vi "Autonomous Independent.vi"() -> ()   [LabVIEW 2017]
doc: "This VI is called when autonomous begins, and will automatically be terminated when autonomous ends. You can carry out timed or sensor driven robot movement independently without needing to return to the caller."
uses:
  Control 1.ctl
  <vilib>/Rock Robotics/WPI/Solenoid/WPI_SolenoidValue.ctl
  <vilib>/Rock Robotics/Network Tables/NT Read String.vi
  <vilib>/Rock Robotics/WPI/Utilities/WPI_GetSetVariantRefNum.vi
  <vilib>/Rock Robotics/Network Tables/NT Write Numeric Array.vi
  <vilib>/Rock Robotics/WPI/RobotDrive/WPI_RobotDriveArcadeDrive_Standard(NoSaturation).vi
  <vilib>/Rock Robotics/WPI/Solenoid/WPI_SolenoidSetEnum.vi
panel:
  out "Current Movement, for debugging":T1 {"Y Joystick Value" scale=1.0..-1.0; "X Joystick Value" scale=-1.0..1.0}
  in  "Array of robot movements":T2(array[cluster])=[{"X Joystick Value"=0.39393939393939403, "Y Joystick Value"=0.0, "Delay (sec)"=1.0, "Movement Name"="turn"}, {"X Joystick Value"=-0.3737373737373737, "Y Joystick Value"=0.0, "Delay (sec)"=1.0, "Movement Name"="turn back"}] {"Y Joystick Value" scale=1.0..-1.0; "X Joystick Value" scale=-1.0..1.0}
  # "Be sure to right-click and choose Data Operations>>Make Current Value default if you want to save the array values with the VI"
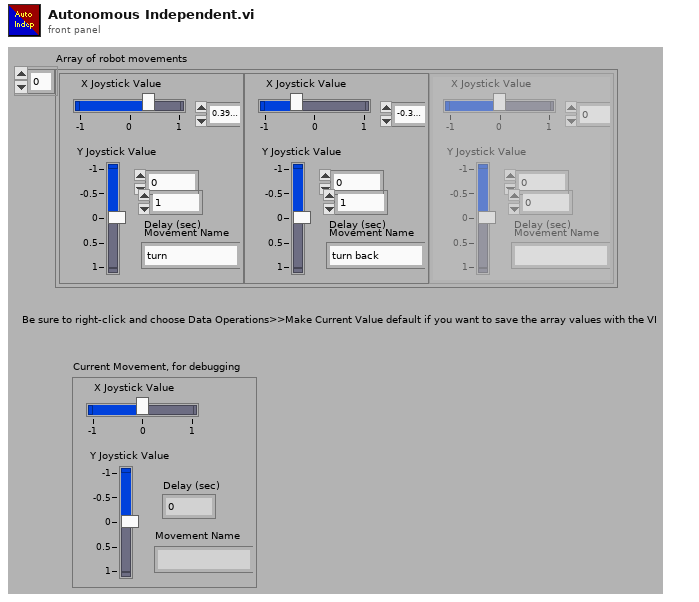
[diagram p1: front panel]
types:
  T1 = cluster{"X Joystick Value":dbl, "Y Joystick Value":dbl, "Delay (sec)":dbl, "Movement Name":string}
  T2 = cluster{"X Joystick Value":dbl, "Y Joystick Value":dbl, "Delay (sec)":dbl, "Movement Name":string}[]
  T3 = typedef "WPI_JoystickDevRef.ctl" = cluster{"Device":T4}
  T4 = typedef "WPI_JoystickDeviceEnum.ctl" = enum16{"USB 0", "USB 1", "USB 2", "USB 3", "USB 4", "USB 5"}
  T5 = typedef "Control 1.ctl" = dbl
  T6 = typedef "WPI_SolenoidValue.ctl" = enum16{"Off", "On", "Forward", "Reverse"}
  T7 = typedef "WPI_RobotDriveDevRef.ctl" = cluster{"DevStatus":errorcluster, "Motors[]":T8[], "Square Inputs":bool, "Max Output":dbl}
  T8 = typedef "WPI_MotorControlDeviceRef.ctl" = cluster{"DeviceStatus":errorcluster, "Type":T9, "PWM":cluster{"PWM Channel":T10, "DeadBand":T11}, "CAN":cluster{"Device Number":u8, "SetOutput VI Ref":variant, "GetOutput VI Ref":variant, "Enable VI Ref":variant, "Disable VI Ref":variant, "Data":variant}, "Invert":bool, "DIO PWM":cluster{"PWM \"Enable\" Channel":T10, "DIOChannel":T12, "PWM Rate":dbl}}
  T9 = typedef "WPI_MotorControlType.ctl" = enum16{"PWM", "CAN", "DIO PWM"}
  T10 = typedef "FPGA_DIOPWMChannel.ctl" = enum8{"PWM 0", "PWM 1", "PWM 2", "PWM 3", "PWM 4", "PWM 5", "PWM 6", "PWM 7", "PWM 8", "PWM 9", "PWM MXP 0", "PWM MXP 1", "PWM MXP 2", "PWM MXP 3", "PWM MXP 4", "PWM MXP 5", "PWM MXP 6", "PWM MXP 7", "PWM MXP 8", "PWM MXP 9", "Invalid"}
  T11 = typedef "WPI_PWMDeadband.ctl" = cluster{"Name":string, "maxPositivePwm":i32, "minPositivePwm":i32, "centerPwm":i32, "maxNegativePwm":i32, "minNegativePwm":i32, "angularRange":u16}
  T12 = typedef "FPGA_DIOChannel.ctl" = enum8{"DIO 0", "DIO 1", "DIO 2", "DIO 3", "DIO 4", "DIO 5", "DIO 6", "DIO 7", "DIO 8", "DIO 9", "DIO MXP 0", "DIO MXP 1", "DIO MXP 2", "DIO MXP 3", "DIO MXP 4", "DIO MXP 5", "DIO MXP 6", "DIO MXP 7", "DIO MXP 8", "DIO MXP 9", "DIO MXP 10", "DIO MXP 11", "DIO MXP 12", "DIO MXP 13", "DIO MXP 14", "DIO MXP 15", "SPI Port CS1", "SPI Port CS2", "SPI Port CS3", "SPI Port MISO", "SPI Port MOSI", "Invalid"}
  T13 = typedef "WPI_SolenoidDevRef.ctl" = cluster{"DevStatus":errorcluster, "Pneumatics Control Module":u8, "Forward Solenoid Channel":T14, "Reverse Solenoid Channel":T14}
  T14 = typedef "WPI_SolenoidChannel.ctl" = enum8{"Solenoid 0", "Solenoid 1", "Solenoid 2", "Solenoid 3", "Solenoid 4", "Solenoid 5", "Solenoid 6", "Solenoid 7", "Invalid"}
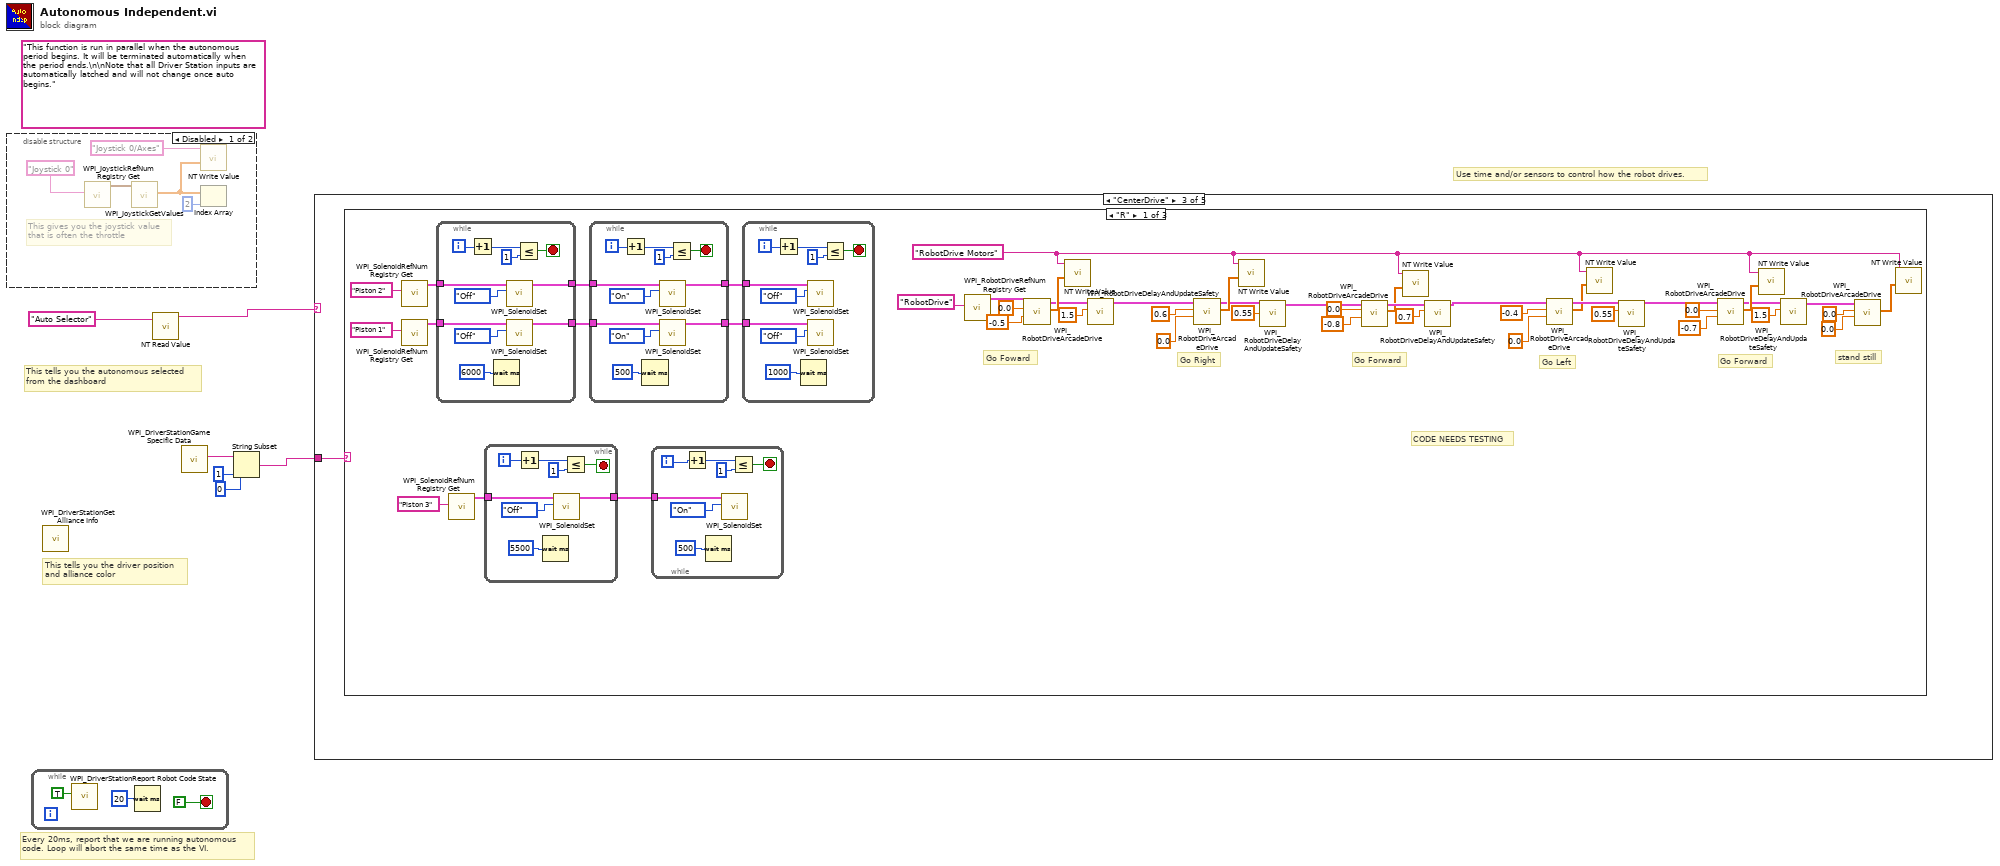
[diagram p0: block diagram]
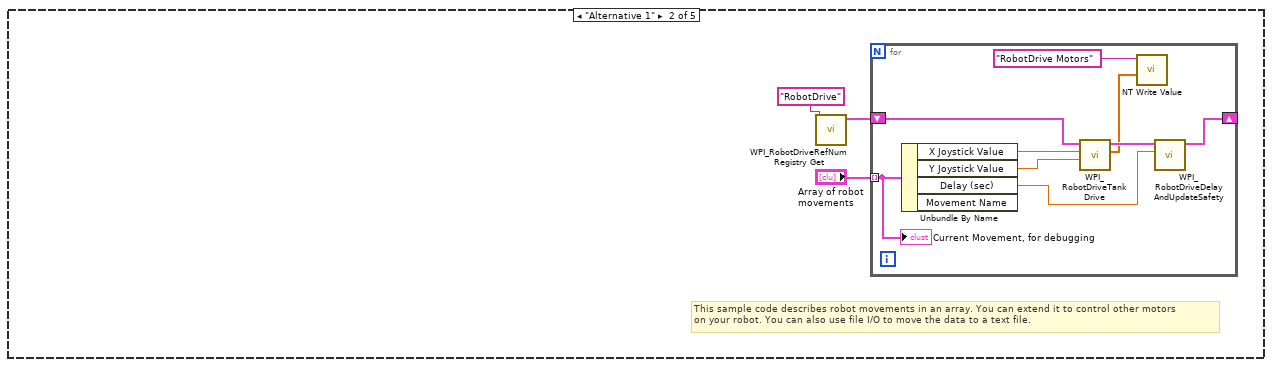
[diagram p4: hidden frame]
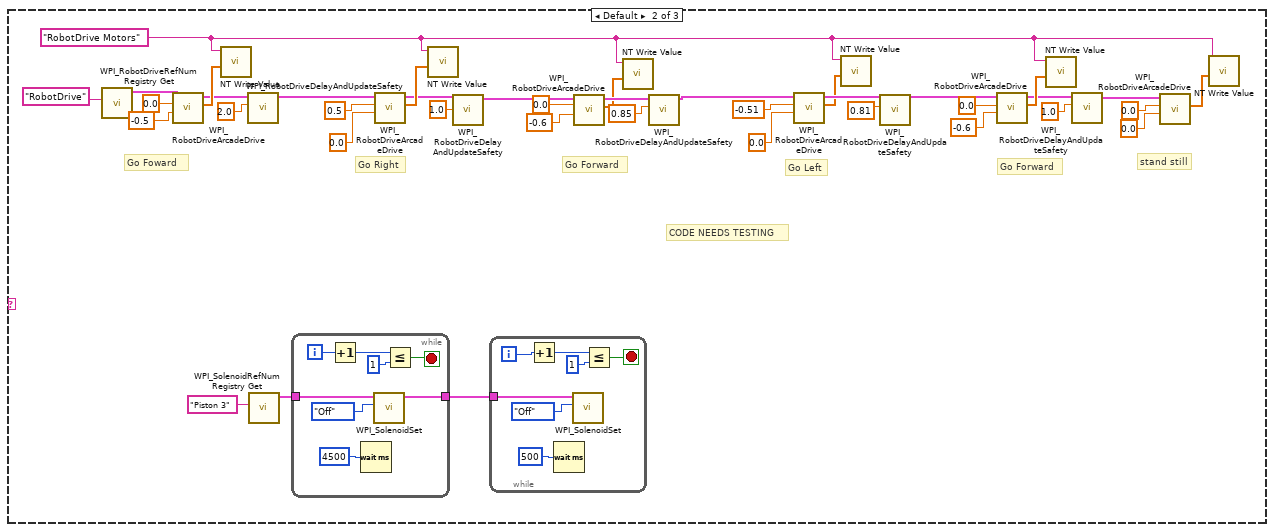
[diagram p5: hidden frame]
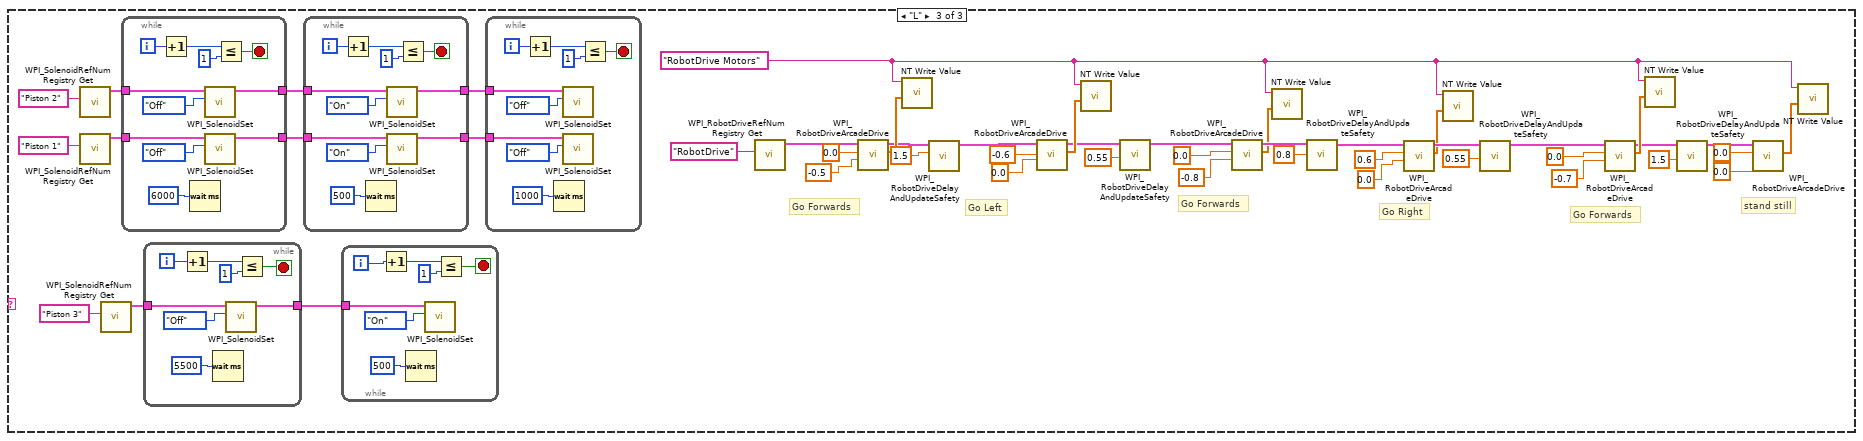
[diagram p6: hidden frame]
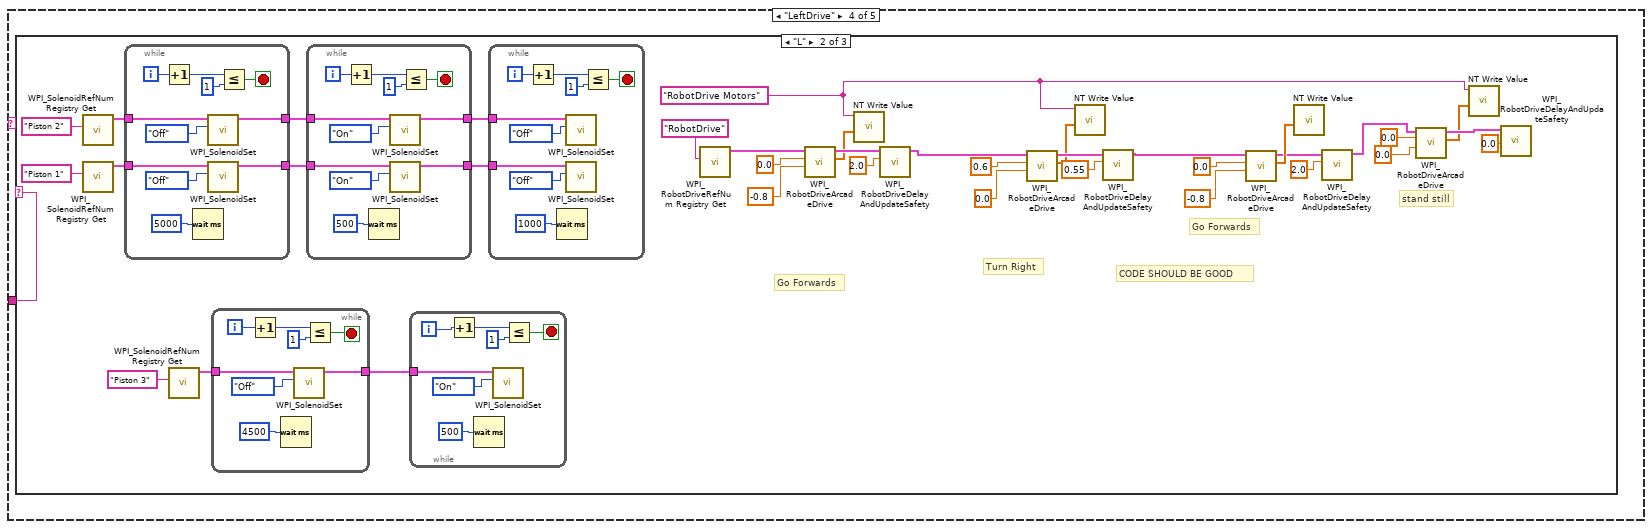
[diagram p7: hidden frame]
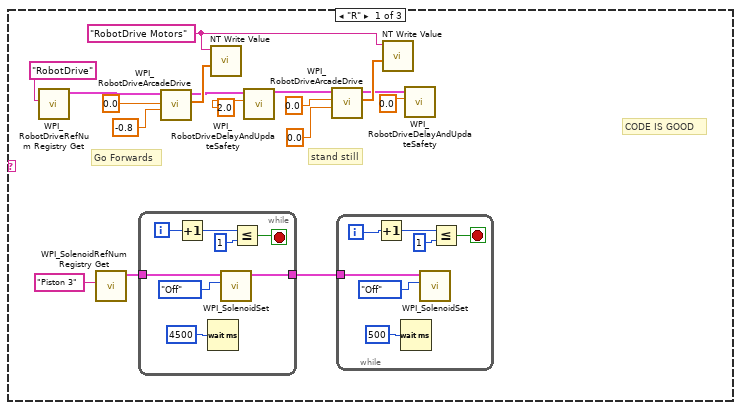
[diagram p8: hidden frame]
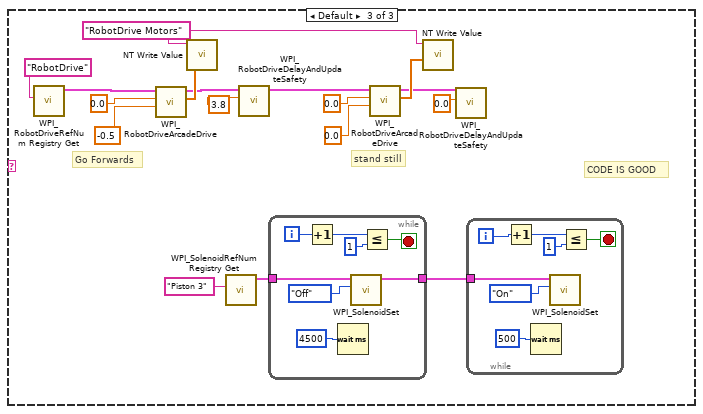
[diagram p9: hidden frame]
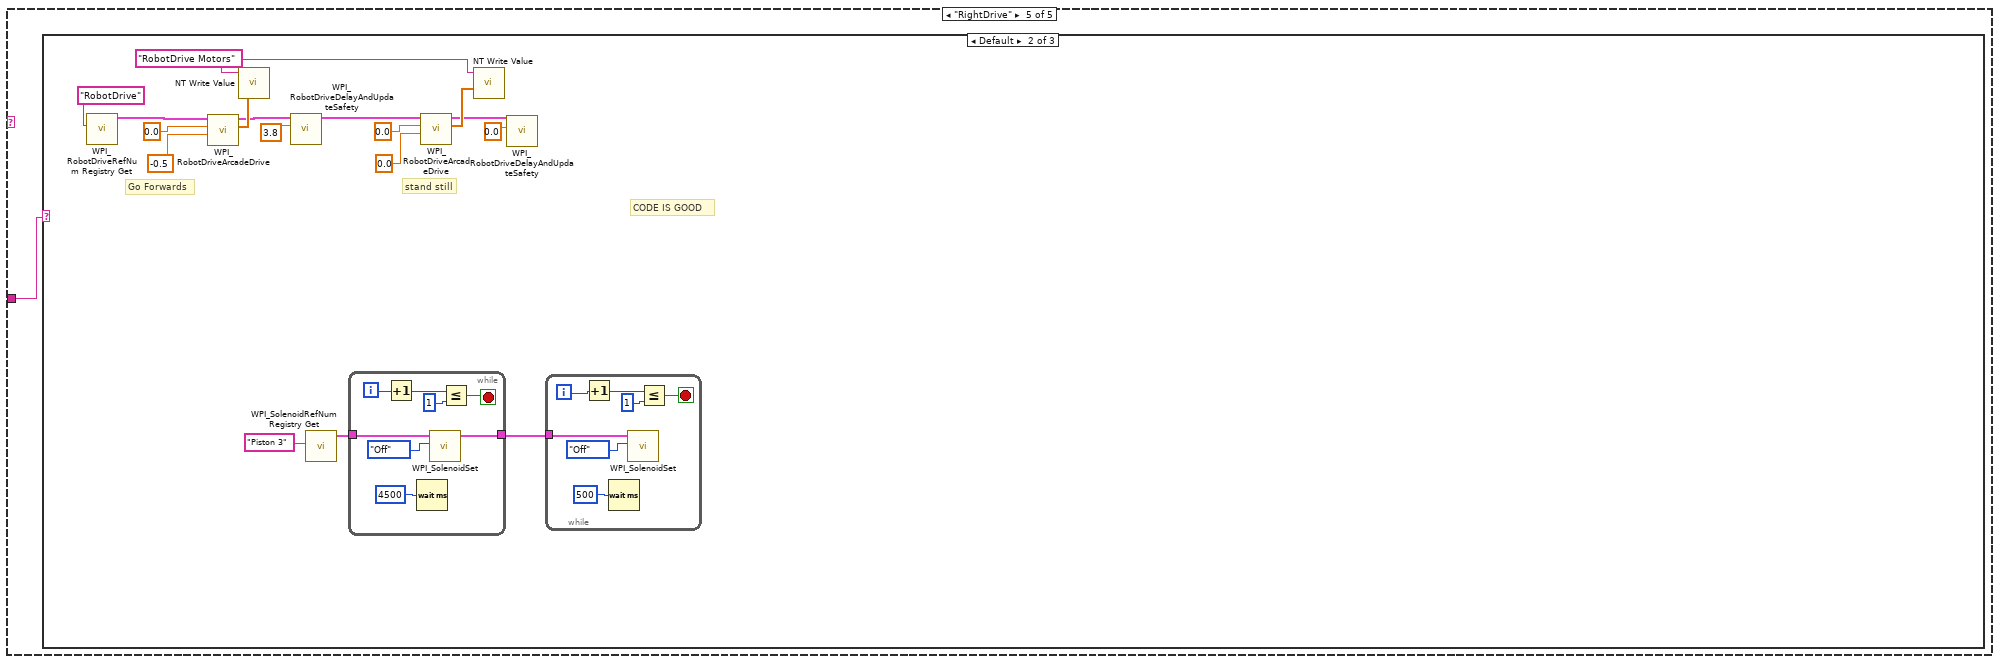
[diagram p10: hidden frame]
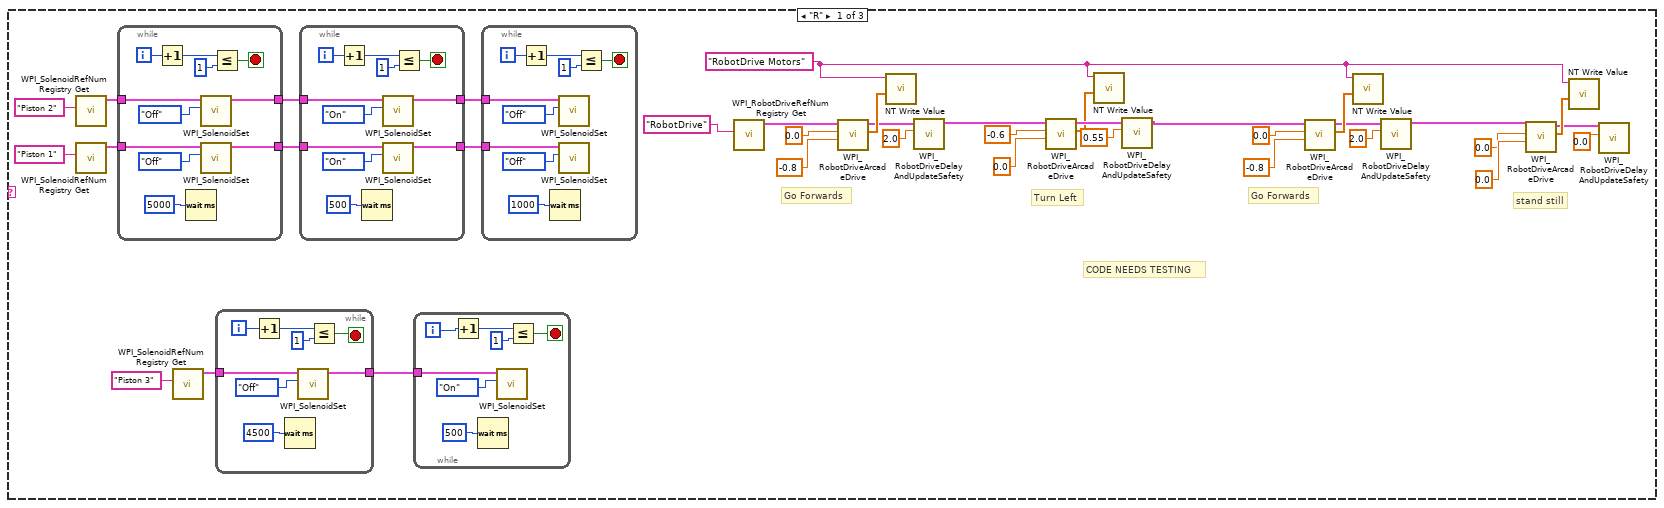
[diagram p11: hidden frame]
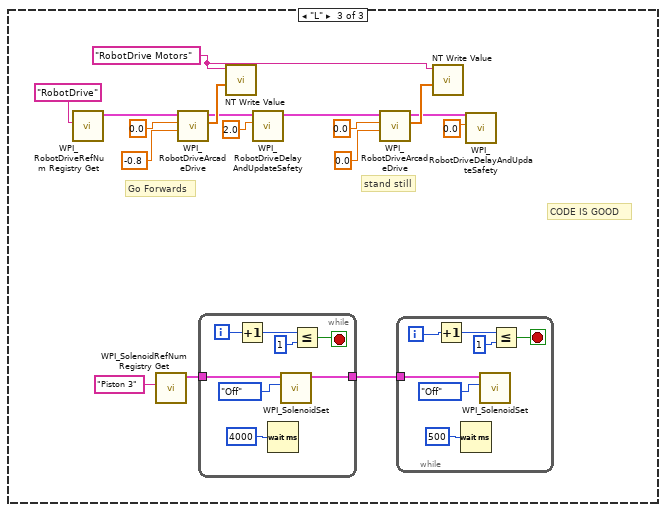
[diagram p12: hidden frame]
diagram:
  (unwired) "This function is run in parallel when the autonomous period begins. It will be terminated automatically when the period ends.\n\nNote that all Driver Station inputs are automatically latched and will not change once auto begins."
  # "This tells you the autonomous selected\nfrom the dashboard"
  # "Every 20ms, report that we are running autonomous\ncode. Loop will abort the same time as the VI."
  # "Use time and/or sensors to control how the robot drives."
  # "This tells you the driver position\nand alliance color"
  n1 = disable-structure shown="Disabled" {
    frame Disabled {
      # "This gives you the joystick value\nthat is often the throttle"
      n2 = call <vilib>:"WPI_JoystickRefNum Registry Get.vi"("refnum name"="Joystick 0") -> ("JoystickDevRef"=w10:T3)  [unwired: 1 in, 9 out]
      n3 = call <vilib>:"WPI_JoystickGetValues.vi"("JoystickDevRef"=w10) -> ("Axes"=w8:dbl[])  [unwired: 6 in, 4 out]
      n4 = call-poly <vilib>:"NT Write Value.vi"("Numeric Array"=w8, "Name"="Joystick 0/Axes") -> ()  [unwired: 9 in, 1 out]
      n5 = Index Array(array=w8, index=2) -> ()  [unwired: 1 out]
    }
    frame Enabled {
    }
  }
  n6 = while {
    stop <- FALSE stop-if-true
    n7 = call <vilib>:"WPI_DriverStationReport Robot Code State.vi"("Autonomous"=TRUE) -> ()  [unwired: 10 in, 1 out]
    n8 = Wait (ms)(milliseconds to wait=u32 20) -> ()  [unwired: 1 out]
  }
  n9 = call <vilib>:"WPI_DriverStationGet Alliance Info.vi"() -> ()  [unwired: 12 out]
  n10 = call-poly <vilib>:"NT Read Value.vi"("Name"="Auto Selector") -> ("String"=w5:string)  [unwired: 9 in, 1 out]
  n11 = call <vilib>:"WPI_DriverStationGame Specific Data.vi"() -> ("Game Specific Data"=w4:string)  [unwired: 11 in]
  n12 = String Subset(string=w4, offset (0)=0, length (rest)=1) -> (substring=w2:string)
  n13 = case shown="\"CenterDrive\"" w5 {
    tunnel: w2 -> [_ _ w27 w268 w416]
    frame Default {
      # "You can put your main auto here, or you can right-click on the case and make any\nother frame be the default case."
      # "This is the frame that will execute if no selection is made, or if it is not recognized"
    }
    frame "Alternative 1" {
      # "This sample code describes robot movements in an array. You can extend it to control other motors\non your robot. You can also use file I/O to move the data to a text file."
      n14 = call <vilib>:"WPI_RobotDriveRefNum Registry Get.vi"("refnum name"="RobotDrive") -> ("RobotDriveDevRef"=w16:T7)  [unwired: 1 in, 9 out]
      n15 = for {
        shift-right: [w24] -> _
        shift-left: w16 -> [w25]
        tunnel: "Array of robot movements" -> [w20] mode=indexing
        n16 = Unbundle By Name(w20) -> ("X Joystick Value"=w23:dbl, "Y Joystick Value"=w22:dbl, "Delay (sec)"=w21:dbl)  [unwired: 1 out]
        n17 = call <vilib>:"WPI_RobotDriveTankDrive.vi"("Right axis value"=w22, "Left axis value"=w23, "RobotDriveDevRef"=w25) -> ("Motor Values"=w18:dbl[], "RobotDriveDevRef"=w26:T7)  [unwired: 6 in, 1 out]
        n18 = call-poly <vilib>:"NT Write Value.vi"("Numeric Array"=w18, "Name"="RobotDrive Motors") -> ()  [unwired: 9 in, 1 out]
        n19 = call <vilib>:"WPI_RobotDriveDelayAndUpdateSafety.vi"("Delay (s)"=w21, "RobotDriveDevRef"=w26) -> ("RobotDriveDevRef 2"=w24:T7)  [unwired: 8 in, 1 out]
        "Current Movement, for debugging" <- w20
      }
    }
    frame "CenterDrive" {
      n20 = case shown="\"R\"" w27 {
        frame "R" {
          w39 = "RobotDrive Motors" ("Name")
          # "CODE NEEDS TESTING"
          # "Go Forward"
          # "Go Left"
          # "Go Forward"
          # "stand still"
          # "Go Right"
          # "Go Foward"
          n21 = call <vilib>:"WPI_SolenoidRefNum Registry Get.vi"("refnum name"="Piston 2") -> ("SolenoidDevRef"=w36:T13)  [unwired: 9 in, 1 out]
          n22 = call <vilib>:"WPI_SolenoidRefNum Registry Get.vi"("refnum name"="Piston 1") -> ("SolenoidDevRef"=w35:T13)  [unwired: 9 in, 1 out]
          n23 = while {
            tunnel: w36 -> [w114]
            tunnel: w35 -> [w112]
            tunnel: [w111] -> w34
            tunnel: [w110] -> w33
            i -> [w120]
            stop <- w118 stop-if-true
            n24 = Increment(x=w120) -> (x+1=w119:i32)
            n25 = Wait (ms)(milliseconds to wait=u32 6000) -> ()  [unwired: 1 out]
            n26 = call-poly <vilib>:"WPI_SolenoidSet.vi"("Value"=WPI_SolenoidValue."Off", "SolenoidDevRef"=w114) -> ("SolenoidDevRef"=w111:T13)  [unwired: 8 in, 1 out]
            n27 = call-poly <vilib>:"WPI_SolenoidSet.vi"("Value"=WPI_SolenoidValue."Off", "SolenoidDevRef"=w112) -> ("SolenoidDevRef"=w110:T13)  [unwired: 8 in, 1 out]
            n28 = Less Or Equal?(x=w119, y=1) -> (x <= y?=w118:bool)
          }
          n29 = call <vilib>:"WPI_SolenoidRefNum Registry Get.vi"("refnum name"="Piston 3") -> ("SolenoidDevRef"=w29:T13)  [unwired: 9 in, 1 out]
          n30 = while {
            tunnel: w29 -> [w83]
            tunnel: [w82] -> w28
            i -> [w84]
            stop <- w85 stop-if-true
            n31 = Increment(x=w84) -> (x+1=w86:i32)
            n32 = Wait (ms)(milliseconds to wait=u32 5500) -> ()  [unwired: 1 out]
            n33 = call-poly <vilib>:"WPI_SolenoidSet.vi"("Value"=WPI_SolenoidValue."Off", "SolenoidDevRef"=w83) -> ("SolenoidDevRef"=w82:T13)  [unwired: 8 in, 1 out]
            n34 = Less Or Equal?(x=w86, y=1) -> (x <= y?=w85:bool)
          }
          n35 = while {
            tunnel: w34 -> [w102]
            tunnel: w33 -> [w101]
            tunnel: [w100] -> w32
            tunnel: [w99] -> w31
            i -> [w106]
            stop <- w105 stop-if-true
            n36 = Increment(x=w106) -> (x+1=w107:i32)
            n37 = Wait (ms)(milliseconds to wait=u32 500) -> ()  [unwired: 1 out]
            n38 = call-poly <vilib>:"WPI_SolenoidSet.vi"("Value"=WPI_SolenoidValue."On", "SolenoidDevRef"=w102) -> ("SolenoidDevRef"=w99:T13)  [unwired: 8 in, 1 out]
            n39 = call-poly <vilib>:"WPI_SolenoidSet.vi"("Value"=WPI_SolenoidValue."On", "SolenoidDevRef"=w101) -> ("SolenoidDevRef"=w100:T13)  [unwired: 8 in, 1 out]
            n40 = Less Or Equal?(x=w107, y=1) -> (x <= y?=w105:bool)
          }
          n41 = while {
            tunnel: w28 -> [w75]
            i -> [w76]
            stop <- w77 stop-if-true
            n42 = Increment(x=w76) -> (x+1=w80:i32)
            n43 = Wait (ms)(milliseconds to wait=u32 500) -> ()  [unwired: 1 out]
            n44 = call-poly <vilib>:"WPI_SolenoidSet.vi"("Value"=WPI_SolenoidValue."On", "SolenoidDevRef"=w75) -> ()  [unwired: 8 in, 2 out]
            n45 = Less Or Equal?(x=w80, y=1) -> (x <= y?=w77:bool)
          }
          n46 = while {
            tunnel: w32 -> [w91]
            tunnel: w31 -> [w90]
            i -> [w95]
            stop <- w94 stop-if-true
            n47 = Increment(x=w95) -> (x+1=w96:i32)
            n48 = Wait (ms)(milliseconds to wait=u32 1000) -> ()  [unwired: 1 out]
            n49 = call-poly <vilib>:"WPI_SolenoidSet.vi"("Value"=WPI_SolenoidValue."Off", "SolenoidDevRef"=w90) -> ()  [unwired: 8 in, 2 out]
            n50 = call-poly <vilib>:"WPI_SolenoidSet.vi"("Value"=WPI_SolenoidValue."Off", "SolenoidDevRef"=w91) -> ()  [unwired: 8 in, 2 out]
            n51 = Less Or Equal?(x=w96, y=1) -> (x <= y?=w94:bool)
          }
          n52 = call <vilib>:"WPI_RobotDriveRefNum Registry Get.vi"("refnum name"="RobotDrive") -> ("RobotDriveDevRef"=w68:T7)  [unwired: 1 in, 9 out]
          n53 = call-poly <vilib>:"WPI_RobotDriveArcadeDrive.vi"("Y axis value"=-0.5 ("X axis value"), "X axis value"=0.0, "RobotDriveDevRef"=w68) -> ("Motor Values"=w74:dbl[], "RobotDriveDevRef"=w71:T7)  [unwired: 6 in, 1 out]
          n54 = call-poly <vilib>:"NT Write Value.vi"("Numeric Array"=w74, "Name"=w39) -> ()  [unwired: 9 in, 1 out]
          n55 = call <vilib>:"WPI_RobotDriveDelayAndUpdateSafety.vi"("Delay (s)"=T5 1.5, "RobotDriveDevRef"=w71) -> ("RobotDriveDevRef 2"=w70:T7)  [unwired: 8 in, 1 out]
          n56 = call-poly <vilib>:"WPI_RobotDriveArcadeDrive.vi"("Y axis value"=0.0 ("X axis value"), "X axis value"=0.6, "RobotDriveDevRef"=w70) -> ("Motor Values"=w73:dbl[], "RobotDriveDevRef"=w69:T7)  [unwired: 6 in, 1 out]
          n57 = call-poly <vilib>:"NT Write Value.vi"("Numeric Array"=w73, "Name"=w39) -> ()  [unwired: 9 in, 1 out]
          n58 = call <vilib>:"WPI_RobotDriveDelayAndUpdateSafety.vi"("Delay (s)"=0.55, "RobotDriveDevRef"=w69) -> ("RobotDriveDevRef 2"=w54:T7)  [unwired: 8 in, 1 out]
          n59 = call-poly <vilib>:"WPI_RobotDriveArcadeDrive.vi"("Y axis value"=-0.8 ("X axis value"), "X axis value"=0.0, "RobotDriveDevRef"=w54) -> ("Motor Values"=w55:dbl[], "RobotDriveDevRef"=w56:T7)  [unwired: 6 in, 1 out]
          n60 = call-poly <vilib>:"NT Write Value.vi"("Numeric Array"=w55, "Name"=w39) -> ()  [unwired: 9 in, 1 out]
          n61 = call <vilib>:"WPI_RobotDriveDelayAndUpdateSafety.vi"("Delay (s)"=T5 0.7, "RobotDriveDevRef"=w56) -> ("RobotDriveDevRef 2"=w48:T7)  [unwired: 8 in, 1 out]
          n62 = call-poly <vilib>:"WPI_RobotDriveArcadeDrive.vi"("Y axis value"=0.0 ("X axis value"), "X axis value"=-0.4, "RobotDriveDevRef"=w48) -> ("Motor Values"=w49:dbl[], "RobotDriveDevRef"=w50:T7)  [unwired: 6 in, 1 out]
          n63 = call-poly <vilib>:"NT Write Value.vi"("Numeric Array"=w49, "Name"=w39) -> ()  [unwired: 9 in, 1 out]
          n64 = call <vilib>:"WPI_RobotDriveDelayAndUpdateSafety.vi"("Delay (s)"=0.55, "RobotDriveDevRef"=w50) -> ("RobotDriveDevRef 2"=w42:T7)  [unwired: 8 in, 1 out]
          n65 = call-poly <vilib>:"WPI_RobotDriveArcadeDrive.vi"("Y axis value"=-0.7 ("X axis value"), "X axis value"=0.0, "RobotDriveDevRef"=w42) -> ("Motor Values"=w47:dbl[], "RobotDriveDevRef"=w46:T7)  [unwired: 6 in, 1 out]
          n66 = call-poly <vilib>:"NT Write Value.vi"("Numeric Array"=w47, "Name"=w39) -> ()  [unwired: 9 in, 1 out]
          n67 = call <vilib>:"WPI_RobotDriveDelayAndUpdateSafety.vi"("Delay (s)"=T5 1.5, "RobotDriveDevRef"=w46) -> ("RobotDriveDevRef 2"=w41:T7)  [unwired: 8 in, 1 out]
          n68 = call-poly <vilib>:"WPI_RobotDriveArcadeDrive.vi"("Y axis value"=0.0 ("X axis value"), "X axis value"=0.0, "RobotDriveDevRef"=w41) -> ("Motor Values"=w72:dbl[])  [unwired: 6 in, 2 out]
          n69 = call-poly <vilib>:"NT Write Value.vi"("Numeric Array"=w72, "Name"=w39) -> ()  [unwired: 9 in, 1 out]
        }
        frame Default {
          w124 = "RobotDrive Motors" ("Name")
          # "CODE NEEDS TESTING"
          # "Go Forward"
          # "Go Left"
          # "Go Forward"
          # "stand still"
          # "Go Right"
          # "Go Foward"
          n70 = call <vilib>:"WPI_RobotDriveRefNum Registry Get.vi"("refnum name"="RobotDrive") -> ("RobotDriveDevRef"=w153:T7)  [unwired: 1 in, 9 out]
          n71 = call-poly <vilib>:"WPI_RobotDriveArcadeDrive.vi"("Y axis value"=-0.5 ("X axis value"), "X axis value"=0.0, "RobotDriveDevRef"=w153) -> ("Motor Values"=w159:dbl[], "RobotDriveDevRef"=w156:T7)  [unwired: 6 in, 1 out]
          n72 = call-poly <vilib>:"NT Write Value.vi"("Numeric Array"=w159, "Name"=w124) -> ()  [unwired: 9 in, 1 out]
          n73 = call <vilib>:"WPI_RobotDriveDelayAndUpdateSafety.vi"("Delay (s)"=T5 2.0, "RobotDriveDevRef"=w156) -> ("RobotDriveDevRef 2"=w155:T7)  [unwired: 8 in, 1 out]
          n74 = call <vilib>:"WPI_SolenoidRefNum Registry Get.vi"("refnum name"="Piston 3") -> ("SolenoidDevRef"=w122:T13)  [unwired: 9 in, 1 out]
          n75 = while {
            tunnel: w122 -> [w168]
            tunnel: [w167] -> w121
            i -> [w169]
            stop <- w170 stop-if-true
            n76 = Increment(x=w169) -> (x+1=w171:i32)
            n77 = Wait (ms)(milliseconds to wait=u32 4500) -> ()  [unwired: 1 out]
            n78 = call-poly <vilib>:"WPI_SolenoidSet.vi"("Value"=WPI_SolenoidValue."Off", "SolenoidDevRef"=w168) -> ("SolenoidDevRef"=w167:T13)  [unwired: 8 in, 1 out]
            n79 = Less Or Equal?(x=w171, y=1) -> (x <= y?=w170:bool)
          }
          n80 = call-poly <vilib>:"WPI_RobotDriveArcadeDrive.vi"("Y axis value"=0.0 ("X axis value"), "X axis value"=0.5, "RobotDriveDevRef"=w155) -> ("Motor Values"=w158:dbl[], "RobotDriveDevRef"=w154:T7)  [unwired: 6 in, 1 out]
          n81 = call-poly <vilib>:"NT Write Value.vi"("Numeric Array"=w158, "Name"=w124) -> ()  [unwired: 9 in, 1 out]
          n82 = call <vilib>:"WPI_RobotDriveDelayAndUpdateSafety.vi"("Delay (s)"=1.0, "RobotDriveDevRef"=w154) -> ("RobotDriveDevRef 2"=w139:T7)  [unwired: 8 in, 1 out]
          n83 = while {
            tunnel: w121 -> [w160]
            i -> [w161]
            stop <- w162 stop-if-true
            n84 = Increment(x=w161) -> (x+1=w165:i32)
            n85 = Wait (ms)(milliseconds to wait=u32 500) -> ()  [unwired: 1 out]
            n86 = call-poly <vilib>:"WPI_SolenoidSet.vi"("Value"=WPI_SolenoidValue."Off", "SolenoidDevRef"=w160) -> ()  [unwired: 8 in, 2 out]
            n87 = Less Or Equal?(x=w165, y=1) -> (x <= y?=w162:bool)
          }
          n88 = call-poly <vilib>:"WPI_RobotDriveArcadeDrive.vi"("Y axis value"=-0.6 ("X axis value"), "X axis value"=0.0, "RobotDriveDevRef"=w139) -> ("Motor Values"=w140:dbl[], "RobotDriveDevRef"=w141:T7)  [unwired: 6 in, 1 out]
          n89 = call-poly <vilib>:"NT Write Value.vi"("Numeric Array"=w140, "Name"=w124) -> ()  [unwired: 9 in, 1 out]
          n90 = call <vilib>:"WPI_RobotDriveDelayAndUpdateSafety.vi"("Delay (s)"=T5 0.85, "RobotDriveDevRef"=w141) -> ("RobotDriveDevRef 2"=w133:T7)  [unwired: 8 in, 1 out]
          n91 = call-poly <vilib>:"WPI_RobotDriveArcadeDrive.vi"("Y axis value"=0.0 ("X axis value"), "X axis value"=-0.51, "RobotDriveDevRef"=w133) -> ("Motor Values"=w134:dbl[], "RobotDriveDevRef"=w135:T7)  [unwired: 6 in, 1 out]
          n92 = call-poly <vilib>:"NT Write Value.vi"("Numeric Array"=w134, "Name"=w124) -> ()  [unwired: 9 in, 1 out]
          n93 = call <vilib>:"WPI_RobotDriveDelayAndUpdateSafety.vi"("Delay (s)"=0.81, "RobotDriveDevRef"=w135) -> ("RobotDriveDevRef 2"=w127:T7)  [unwired: 8 in, 1 out]
          n94 = call-poly <vilib>:"WPI_RobotDriveArcadeDrive.vi"("Y axis value"=-0.6 ("X axis value"), "X axis value"=0.0, "RobotDriveDevRef"=w127) -> ("Motor Values"=w132:dbl[], "RobotDriveDevRef"=w131:T7)  [unwired: 6 in, 1 out]
          n95 = call-poly <vilib>:"NT Write Value.vi"("Numeric Array"=w132, "Name"=w124) -> ()  [unwired: 9 in, 1 out]
          n96 = call <vilib>:"WPI_RobotDriveDelayAndUpdateSafety.vi"("Delay (s)"=T5 1.0, "RobotDriveDevRef"=w131) -> ("RobotDriveDevRef 2"=w126:T7)  [unwired: 8 in, 1 out]
          n97 = call-poly <vilib>:"WPI_RobotDriveArcadeDrive.vi"("Y axis value"=0.0 ("X axis value"), "X axis value"=0.0, "RobotDriveDevRef"=w126) -> ("Motor Values"=w157:dbl[])  [unwired: 6 in, 2 out]
          n98 = call-poly <vilib>:"NT Write Value.vi"("Numeric Array"=w157, "Name"=w124) -> ()  [unwired: 9 in, 1 out]
        }
        frame "L" {
          w186 = "RobotDrive Motors" ("Name")
          # "Go Forwards"
          # "Go Right"
          # "Go Forwards"
          # "stand still"
          # "Go Left"
          # "Go Forwards"
          n99 = call <vilib>:"WPI_SolenoidRefNum Registry Get.vi"("refnum name"="Piston 2") -> ("SolenoidDevRef"=w183:T13)  [unwired: 9 in, 1 out]
          n100 = call <vilib>:"WPI_SolenoidRefNum Registry Get.vi"("refnum name"="Piston 1") -> ("SolenoidDevRef"=w182:T13)  [unwired: 9 in, 1 out]
          n101 = call <vilib>:"WPI_SolenoidRefNum Registry Get.vi"("refnum name"="Piston 3") -> ("SolenoidDevRef"=w176:T13)  [unwired: 9 in, 1 out]
          n102 = while {
            tunnel: w183 -> [w261]
            tunnel: w182 -> [w259]
            tunnel: [w258] -> w181
            tunnel: [w257] -> w180
            i -> [w267]
            stop <- w265 stop-if-true
            n103 = Increment(x=w267) -> (x+1=w266:i32)
            n104 = Wait (ms)(milliseconds to wait=u32 6000) -> ()  [unwired: 1 out]
            n105 = call-poly <vilib>:"WPI_SolenoidSet.vi"("Value"=WPI_SolenoidValue."Off", "SolenoidDevRef"=w261) -> ("SolenoidDevRef"=w258:T13)  [unwired: 8 in, 1 out]
            n106 = call-poly <vilib>:"WPI_SolenoidSet.vi"("Value"=WPI_SolenoidValue."Off", "SolenoidDevRef"=w259) -> ("SolenoidDevRef"=w257:T13)  [unwired: 8 in, 1 out]
            n107 = Less Or Equal?(x=w266, y=1) -> (x <= y?=w265:bool)
          }
          n108 = while {
            tunnel: w176 -> [w230]
            tunnel: [w229] -> w175
            i -> [w231]
            stop <- w232 stop-if-true
            n109 = Increment(x=w231) -> (x+1=w233:i32)
            n110 = Wait (ms)(milliseconds to wait=u32 5500) -> ()  [unwired: 1 out]
            n111 = call-poly <vilib>:"WPI_SolenoidSet.vi"("Value"=WPI_SolenoidValue."Off", "SolenoidDevRef"=w230) -> ("SolenoidDevRef"=w229:T13)  [unwired: 8 in, 1 out]
            n112 = Less Or Equal?(x=w233, y=1) -> (x <= y?=w232:bool)
          }
          n113 = while {
            tunnel: w181 -> [w249]
            tunnel: w180 -> [w248]
            tunnel: [w247] -> w179
            tunnel: [w246] -> w178
            i -> [w253]
            stop <- w252 stop-if-true
            n114 = Increment(x=w253) -> (x+1=w254:i32)
            n115 = Wait (ms)(milliseconds to wait=u32 500) -> ()  [unwired: 1 out]
            n116 = call-poly <vilib>:"WPI_SolenoidSet.vi"("Value"=WPI_SolenoidValue."On", "SolenoidDevRef"=w249) -> ("SolenoidDevRef"=w246:T13)  [unwired: 8 in, 1 out]
            n117 = call-poly <vilib>:"WPI_SolenoidSet.vi"("Value"=WPI_SolenoidValue."On", "SolenoidDevRef"=w248) -> ("SolenoidDevRef"=w247:T13)  [unwired: 8 in, 1 out]
            n118 = Less Or Equal?(x=w254, y=1) -> (x <= y?=w252:bool)
          }
          n119 = while {
            tunnel: w175 -> [w222]
            i -> [w223]
            stop <- w224 stop-if-true
            n120 = Increment(x=w223) -> (x+1=w227:i32)
            n121 = Wait (ms)(milliseconds to wait=u32 500) -> ()  [unwired: 1 out]
            n122 = call-poly <vilib>:"WPI_SolenoidSet.vi"("Value"=WPI_SolenoidValue."On", "SolenoidDevRef"=w222) -> ()  [unwired: 8 in, 2 out]
            n123 = Less Or Equal?(x=w227, y=1) -> (x <= y?=w224:bool)
          }
          n124 = while {
            tunnel: w179 -> [w238]
            tunnel: w178 -> [w237]
            i -> [w242]
            stop <- w241 stop-if-true
            n125 = Increment(x=w242) -> (x+1=w243:i32)
            n126 = Wait (ms)(milliseconds to wait=u32 1000) -> ()  [unwired: 1 out]
            n127 = call-poly <vilib>:"WPI_SolenoidSet.vi"("Value"=WPI_SolenoidValue."Off", "SolenoidDevRef"=w237) -> ()  [unwired: 8 in, 2 out]
            n128 = call-poly <vilib>:"WPI_SolenoidSet.vi"("Value"=WPI_SolenoidValue."Off", "SolenoidDevRef"=w238) -> ()  [unwired: 8 in, 2 out]
            n129 = Less Or Equal?(x=w243, y=1) -> (x <= y?=w241:bool)
          }
          n130 = call <vilib>:"WPI_RobotDriveRefNum Registry Get.vi"("refnum name"="RobotDrive") -> ("RobotDriveDevRef"=w215:T7)  [unwired: 1 in, 9 out]
          n131 = call-poly <vilib>:"WPI_RobotDriveArcadeDrive.vi"("Y axis value"=-0.5 ("X axis value"), "X axis value"=0.0, "RobotDriveDevRef"=w215) -> ("Motor Values"=w221:dbl[], "RobotDriveDevRef"=w218:T7)  [unwired: 6 in, 1 out]
          n132 = call-poly <vilib>:"NT Write Value.vi"("Numeric Array"=w221, "Name"=w186) -> ()  [unwired: 9 in, 1 out]
          n133 = call <vilib>:"WPI_RobotDriveDelayAndUpdateSafety.vi"("Delay (s)"=T5 1.5, "RobotDriveDevRef"=w218) -> ("RobotDriveDevRef 2"=w217:T7)  [unwired: 8 in, 1 out]
          n134 = call-poly <vilib>:"WPI_RobotDriveArcadeDrive.vi"("Y axis value"=0.0 ("X axis value"), "X axis value"=-0.6, "RobotDriveDevRef"=w217) -> ("Motor Values"=w220:dbl[], "RobotDriveDevRef"=w216:T7)  [unwired: 6 in, 1 out]
          n135 = call-poly <vilib>:"NT Write Value.vi"("Numeric Array"=w220, "Name"=w186) -> ()  [unwired: 9 in, 1 out]
          n136 = call <vilib>:"WPI_RobotDriveDelayAndUpdateSafety.vi"("Delay (s)"=0.55, "RobotDriveDevRef"=w216) -> ("RobotDriveDevRef 2"=w201:T7)  [unwired: 8 in, 1 out]
          n137 = call-poly <vilib>:"WPI_RobotDriveArcadeDrive.vi"("Y axis value"=-0.8 ("X axis value"), "X axis value"=0.0, "RobotDriveDevRef"=w201) -> ("Motor Values"=w202:dbl[], "RobotDriveDevRef"=w203:T7)  [unwired: 6 in, 1 out]
          n138 = call-poly <vilib>:"NT Write Value.vi"("Numeric Array"=w202, "Name"=w186) -> ()  [unwired: 9 in, 1 out]
          n139 = call <vilib>:"WPI_RobotDriveDelayAndUpdateSafety.vi"("Delay (s)"=T5 0.8, "RobotDriveDevRef"=w203) -> ("RobotDriveDevRef 2"=w195:T7)  [unwired: 8 in, 1 out]
          n140 = call-poly <vilib>:"WPI_RobotDriveArcadeDrive.vi"("Y axis value"=0.0 ("X axis value"), "X axis value"=0.6, "RobotDriveDevRef"=w195) -> ("Motor Values"=w196:dbl[], "RobotDriveDevRef"=w197:T7)  [unwired: 6 in, 1 out]
          n141 = call-poly <vilib>:"NT Write Value.vi"("Numeric Array"=w196, "Name"=w186) -> ()  [unwired: 9 in, 1 out]
          n142 = call <vilib>:"WPI_RobotDriveDelayAndUpdateSafety.vi"("Delay (s)"=0.55, "RobotDriveDevRef"=w197) -> ("RobotDriveDevRef 2"=w189:T7)  [unwired: 8 in, 1 out]
          n143 = call-poly <vilib>:"WPI_RobotDriveArcadeDrive.vi"("Y axis value"=-0.7 ("X axis value"), "X axis value"=0.0, "RobotDriveDevRef"=w189) -> ("Motor Values"=w194:dbl[], "RobotDriveDevRef"=w193:T7)  [unwired: 6 in, 1 out]
          n144 = call-poly <vilib>:"NT Write Value.vi"("Numeric Array"=w194, "Name"=w186) -> ()  [unwired: 9 in, 1 out]
          n145 = call <vilib>:"WPI_RobotDriveDelayAndUpdateSafety.vi"("Delay (s)"=T5 1.5, "RobotDriveDevRef"=w193) -> ("RobotDriveDevRef 2"=w188:T7)  [unwired: 8 in, 1 out]
          n146 = call-poly <vilib>:"WPI_RobotDriveArcadeDrive.vi"("Y axis value"=0.0 ("X axis value"), "X axis value"=0.0, "RobotDriveDevRef"=w188) -> ("Motor Values"=w219:dbl[])  [unwired: 6 in, 2 out]
          n147 = call-poly <vilib>:"NT Write Value.vi"("Numeric Array"=w219, "Name"=w186) -> ()  [unwired: 9 in, 1 out]
        }
      }
    }
    frame "LeftDrive" {
      n148 = case shown="\"L\"" w268 {
        frame "R" {
          w275 = "RobotDrive Motors" ("Name")
          # "CODE IS GOOD"
          # "stand still"
          # "Go Forwards"
          n149 = call <vilib>:"WPI_RobotDriveRefNum Registry Get.vi"("refnum name"="RobotDrive") -> ("RobotDriveDevRef"=w280:T7)  [unwired: 1 in, 9 out]
          n150 = call <vilib>:"WPI_SolenoidRefNum Registry Get.vi"("refnum name"="Piston 3") -> ("SolenoidDevRef"=w270:T13)  [unwired: 9 in, 1 out]
          n151 = while {
            tunnel: w270 -> [w294]
            tunnel: [w293] -> w269
            i -> [w295]
            stop <- w296 stop-if-true
            n152 = Increment(x=w295) -> (x+1=w297:i32)
            n153 = Wait (ms)(milliseconds to wait=u32 4500) -> ()  [unwired: 1 out]
            n154 = call-poly <vilib>:"WPI_SolenoidSet.vi"("Value"=WPI_SolenoidValue."Off", "SolenoidDevRef"=w294) -> ("SolenoidDevRef"=w293:T13)  [unwired: 8 in, 1 out]
            n155 = Less Or Equal?(x=w297, y=1) -> (x <= y?=w296:bool)
          }
          n156 = call-poly <vilib>:"WPI_RobotDriveArcadeDrive.vi"("Y axis value"=-0.8 ("X axis value"), "X axis value"=0.0, "RobotDriveDevRef"=w280) -> ("Motor Values"=w285:dbl[], "RobotDriveDevRef"=w283:T7)  [unwired: 6 in, 1 out]
          n157 = call-poly <vilib>:"NT Write Value.vi"("Numeric Array"=w285, "Name"=w275) -> ()  [unwired: 9 in, 1 out]
          n158 = call <vilib>:"WPI_RobotDriveDelayAndUpdateSafety.vi"("Delay (s)"=T5 2.0, "RobotDriveDevRef"=w283) -> ("RobotDriveDevRef 2"=w282:T7)  [unwired: 8 in, 1 out]
          n159 = call-poly <vilib>:"WPI_RobotDriveArcadeDrive.vi"("Y axis value"=0.0 ("X axis value"), "X axis value"=0.0, "RobotDriveDevRef"=w282) -> ("Motor Values"=w284:dbl[], "RobotDriveDevRef"=w281:T7)  [unwired: 6 in, 1 out]
          n160 = while {
            tunnel: w269 -> [w286]
            i -> [w287]
            stop <- w288 stop-if-true
            n161 = Increment(x=w287) -> (x+1=w291:i32)
            n162 = Wait (ms)(milliseconds to wait=u32 500) -> ()  [unwired: 1 out]
            n163 = call-poly <vilib>:"WPI_SolenoidSet.vi"("Value"=WPI_SolenoidValue."Off", "SolenoidDevRef"=w286) -> ()  [unwired: 8 in, 2 out]
            n164 = Less Or Equal?(x=w291, y=1) -> (x <= y?=w288:bool)
          }
          n165 = call-poly <vilib>:"NT Write Value.vi"("Numeric Array"=w284, "Name"=w275) -> ()  [unwired: 9 in, 1 out]
          n166 = call <vilib>:"WPI_RobotDriveDelayAndUpdateSafety.vi"("Delay (s)"=0.0, "RobotDriveDevRef"=w281) -> ()  [unwired: 8 in, 2 out]
        }
        frame "L" {
          w308 = "RobotDrive Motors" ("Name")
          # "Go Forwards"
          # "Turn Right"
          # "CODE SHOULD BE GOOD"
          # "stand still"
          # "Go Forwards"
          n167 = call <vilib>:"WPI_SolenoidRefNum Registry Get.vi"("refnum name"="Piston 2") -> ("SolenoidDevRef"=w324:T13)  [unwired: 9 in, 1 out]
          n168 = call <vilib>:"WPI_SolenoidRefNum Registry Get.vi"("refnum name"="Piston 1") -> ("SolenoidDevRef"=w323:T13)  [unwired: 9 in, 1 out]
          n169 = while {
            tunnel: w324 -> [w377]
            tunnel: w323 -> [w375]
            tunnel: [w374] -> w322
            tunnel: [w373] -> w321
            i -> [w383]
            stop <- w381 stop-if-true
            n170 = Increment(x=w383) -> (x+1=w382:i32)
            n171 = Wait (ms)(milliseconds to wait=u32 5000) -> ()  [unwired: 1 out]
            n172 = call-poly <vilib>:"WPI_SolenoidSet.vi"("Value"=WPI_SolenoidValue."Off", "SolenoidDevRef"=w377) -> ("SolenoidDevRef"=w374:T13)  [unwired: 8 in, 1 out]
            n173 = call-poly <vilib>:"WPI_SolenoidSet.vi"("Value"=WPI_SolenoidValue."Off", "SolenoidDevRef"=w375) -> ("SolenoidDevRef"=w373:T13)  [unwired: 8 in, 1 out]
            n174 = Less Or Equal?(x=w382, y=1) -> (x <= y?=w381:bool)
          }
          n175 = call <vilib>:"WPI_SolenoidRefNum Registry Get.vi"("refnum name"="Piston 3") -> ("SolenoidDevRef"=w316:T13)  [unwired: 9 in, 1 out]
          n176 = while {
            tunnel: w316 -> [w346]
            tunnel: [w345] -> w315
            i -> [w347]
            stop <- w348 stop-if-true
            n177 = Increment(x=w347) -> (x+1=w349:i32)
            n178 = Wait (ms)(milliseconds to wait=u32 4500) -> ()  [unwired: 1 out]
            n179 = call-poly <vilib>:"WPI_SolenoidSet.vi"("Value"=WPI_SolenoidValue."Off", "SolenoidDevRef"=w346) -> ("SolenoidDevRef"=w345:T13)  [unwired: 8 in, 1 out]
            n180 = Less Or Equal?(x=w349, y=1) -> (x <= y?=w348:bool)
          }
          n181 = while {
            tunnel: w322 -> [w365]
            tunnel: w321 -> [w364]
            tunnel: [w363] -> w320
            tunnel: [w362] -> w319
            i -> [w369]
            stop <- w368 stop-if-true
            n182 = Increment(x=w369) -> (x+1=w370:i32)
            n183 = Wait (ms)(milliseconds to wait=u32 500) -> ()  [unwired: 1 out]
            n184 = call-poly <vilib>:"WPI_SolenoidSet.vi"("Value"=WPI_SolenoidValue."On", "SolenoidDevRef"=w365) -> ("SolenoidDevRef"=w362:T13)  [unwired: 8 in, 1 out]
            n185 = call-poly <vilib>:"WPI_SolenoidSet.vi"("Value"=WPI_SolenoidValue."On", "SolenoidDevRef"=w364) -> ("SolenoidDevRef"=w363:T13)  [unwired: 8 in, 1 out]
            n186 = Less Or Equal?(x=w370, y=1) -> (x <= y?=w368:bool)
          }
          n187 = while {
            tunnel: w315 -> [w338]
            i -> [w339]
            stop <- w340 stop-if-true
            n188 = Increment(x=w339) -> (x+1=w343:i32)
            n189 = Wait (ms)(milliseconds to wait=u32 500) -> ()  [unwired: 1 out]
            n190 = call-poly <vilib>:"WPI_SolenoidSet.vi"("Value"=WPI_SolenoidValue."On", "SolenoidDevRef"=w338) -> ()  [unwired: 8 in, 2 out]
            n191 = Less Or Equal?(x=w343, y=1) -> (x <= y?=w340:bool)
          }
          n192 = while {
            tunnel: w320 -> [w354]
            tunnel: w319 -> [w353]
            i -> [w358]
            stop <- w357 stop-if-true
            n193 = Increment(x=w358) -> (x+1=w359:i32)
            n194 = Wait (ms)(milliseconds to wait=u32 1000) -> ()  [unwired: 1 out]
            n195 = call-poly <vilib>:"WPI_SolenoidSet.vi"("Value"=WPI_SolenoidValue."Off", "SolenoidDevRef"=w353) -> ()  [unwired: 8 in, 2 out]
            n196 = call-poly <vilib>:"WPI_SolenoidSet.vi"("Value"=WPI_SolenoidValue."Off", "SolenoidDevRef"=w354) -> ()  [unwired: 8 in, 2 out]
            n197 = Less Or Equal?(x=w359, y=1) -> (x <= y?=w357:bool)
          }
          n198 = call <vilib>:"WPI_RobotDriveRefNum Registry Get.vi"("refnum name"="RobotDrive") -> ("RobotDriveDevRef"=w337:T7)  [unwired: 1 in, 9 out]
          n199 = call-poly <vilib>:"WPI_RobotDriveArcadeDrive.vi"("Y axis value"=-0.8 ("X axis value"), "X axis value"=0.0, "RobotDriveDevRef"=w337) -> ("Motor Values"=w333:dbl[], "RobotDriveDevRef"=w335:T7)  [unwired: 6 in, 1 out]
          n200 = call-poly <vilib>:"NT Write Value.vi"("Numeric Array"=w333, "Name"=w308) -> ()  [unwired: 9 in, 1 out]
          n201 = call <vilib>:"WPI_RobotDriveDelayAndUpdateSafety.vi"("Delay (s)"=T5 2.0, "RobotDriveDevRef"=w335) -> ("RobotDriveDevRef 2"=w309:T7)  [unwired: 8 in, 1 out]
          n202 = call-poly <vilib>:"WPI_RobotDriveArcadeDrive.vi"("Y axis value"=0.0 ("X axis value"), "X axis value"=0.6, "RobotDriveDevRef"=w309) -> ("Motor Values"=w310:dbl[], "RobotDriveDevRef"=w311:T7)  [unwired: 6 in, 1 out]
          n203 = call-poly <vilib>:"NT Write Value.vi"("Numeric Array"=w310, "Name"=w308) -> ()  [unwired: 9 in, 1 out]
          n204 = call <vilib>:"WPI_RobotDriveDelayAndUpdateSafety.vi"("Delay (s)"=T5 0.55, "RobotDriveDevRef"=w311) -> ("RobotDriveDevRef 2"=w302:T7)  [unwired: 8 in, 1 out]
          n205 = call-poly <vilib>:"WPI_RobotDriveArcadeDrive.vi"("Y axis value"=-0.8 ("X axis value"), "X axis value"=0.0, "RobotDriveDevRef"=w302) -> ("Motor Values"=w307:dbl[], "RobotDriveDevRef"=w306:T7)  [unwired: 6 in, 1 out]
          n206 = call-poly <vilib>:"NT Write Value.vi"("Numeric Array"=w307) -> ()  [unwired: 10 in, 1 out]
          n207 = call <vilib>:"WPI_RobotDriveDelayAndUpdateSafety.vi"("Delay (s)"=T5 2.0, "RobotDriveDevRef"=w306) -> ("RobotDriveDevRef 2"=w301:T7)  [unwired: 8 in, 1 out]
          n208 = call-poly <vilib>:"WPI_RobotDriveArcadeDrive.vi"("Y axis value"=0.0 ("X axis value"), "X axis value"=0.0, "RobotDriveDevRef"=w301) -> ("Motor Values"=w334:dbl[], "RobotDriveDevRef"=w336:T7)  [unwired: 6 in, 1 out]
          n209 = call-poly <vilib>:"NT Write Value.vi"("Numeric Array"=w334, "Name"=w308) -> ()  [unwired: 9 in, 1 out]
          n210 = call <vilib>:"WPI_RobotDriveDelayAndUpdateSafety.vi"("Delay (s)"=0.0, "RobotDriveDevRef"=w336) -> ()  [unwired: 8 in, 2 out]
        }
        frame Default {
          w390 = "RobotDrive Motors" ("Name")
          # "CODE IS GOOD"
          # "stand still"
          # "Go Forwards"
          n211 = call <vilib>:"WPI_RobotDriveRefNum Registry Get.vi"("refnum name"="RobotDrive") -> ("RobotDriveDevRef"=w395:T7)  [unwired: 1 in, 9 out]
          n212 = call-poly <vilib>:"WPI_RobotDriveArcadeDrive.vi"("Y axis value"=-0.5 ("X axis value"), "X axis value"=0.0, "RobotDriveDevRef"=w395) -> ("Motor Values"=w400:dbl[], "RobotDriveDevRef"=w398:T7)  [unwired: 6 in, 1 out]
          n213 = call-poly <vilib>:"NT Write Value.vi"("Numeric Array"=w400, "Name"=w390) -> ()  [unwired: 9 in, 1 out]
          n214 = call <vilib>:"WPI_SolenoidRefNum Registry Get.vi"("refnum name"="Piston 3") -> ("SolenoidDevRef"=w385:T13)  [unwired: 9 in, 1 out]
          n215 = call <vilib>:"WPI_RobotDriveDelayAndUpdateSafety.vi"("Delay (s)"=T5 3.8, "RobotDriveDevRef"=w398) -> ("RobotDriveDevRef 2"=w397:T7)  [unwired: 8 in, 1 out]
          n216 = while {
            tunnel: w385 -> [w409]
            tunnel: [w408] -> w384
            i -> [w410]
            stop <- w411 stop-if-true
            n217 = Increment(x=w410) -> (x+1=w412:i32)
            n218 = Wait (ms)(milliseconds to wait=u32 4500) -> ()  [unwired: 1 out]
            n219 = call-poly <vilib>:"WPI_SolenoidSet.vi"("Value"=WPI_SolenoidValue."Off", "SolenoidDevRef"=w409) -> ("SolenoidDevRef"=w408:T13)  [unwired: 8 in, 1 out]
            n220 = Less Or Equal?(x=w412, y=1) -> (x <= y?=w411:bool)
          }
          n221 = call-poly <vilib>:"WPI_RobotDriveArcadeDrive.vi"("Y axis value"=0.0 ("X axis value"), "X axis value"=0.0, "RobotDriveDevRef"=w397) -> ("Motor Values"=w399:dbl[], "RobotDriveDevRef"=w396:T7)  [unwired: 6 in, 1 out]
          n222 = call-poly <vilib>:"NT Write Value.vi"("Numeric Array"=w399, "Name"=w390) -> ()  [unwired: 9 in, 1 out]
          n223 = call <vilib>:"WPI_RobotDriveDelayAndUpdateSafety.vi"("Delay (s)"=0.0, "RobotDriveDevRef"=w396) -> ()  [unwired: 8 in, 2 out]
          n224 = while {
            tunnel: w384 -> [w401]
            i -> [w402]
            stop <- w403 stop-if-true
            n225 = Increment(x=w402) -> (x+1=w406:i32)
            n226 = Wait (ms)(milliseconds to wait=u32 500) -> ()  [unwired: 1 out]
            n227 = call-poly <vilib>:"WPI_SolenoidSet.vi"("Value"=WPI_SolenoidValue."On", "SolenoidDevRef"=w401) -> ()  [unwired: 8 in, 2 out]
            n228 = Less Or Equal?(x=w406, y=1) -> (x <= y?=w403:bool)
          }
        }
      }
    }
    frame "RightDrive" {
      n229 = case shown="Default" w416 {
        frame "R" {
          w417 = "RobotDrive Motors" ("Name")
          w429 = 0.0 ("Delay (s)")
          # "Go Forwards"
          # "CODE NEEDS TESTING"
          # "Turn Left"
          # "stand still"
          # "Go Forwards"
          n230 = call <vilib>:"WPI_SolenoidRefNum Registry Get.vi"("refnum name"="Piston 2") -> ("SolenoidDevRef"=w440:T13)  [unwired: 9 in, 1 out]
          n231 = call <vilib>:"WPI_SolenoidRefNum Registry Get.vi"("refnum name"="Piston 1") -> ("SolenoidDevRef"=w439:T13)  [unwired: 9 in, 1 out]
          n232 = while {
            tunnel: w440 -> [w493]
            tunnel: w439 -> [w491]
            tunnel: [w490] -> w438
            tunnel: [w489] -> w437
            i -> [w499]
            stop <- w497 stop-if-true
            n233 = Increment(x=w499) -> (x+1=w498:i32)
            n234 = Wait (ms)(milliseconds to wait=u32 5000) -> ()  [unwired: 1 out]
            n235 = call-poly <vilib>:"WPI_SolenoidSet.vi"("Value"=WPI_SolenoidValue."Off", "SolenoidDevRef"=w493) -> ("SolenoidDevRef"=w490:T13)  [unwired: 8 in, 1 out]
            n236 = call-poly <vilib>:"WPI_SolenoidSet.vi"("Value"=WPI_SolenoidValue."Off", "SolenoidDevRef"=w491) -> ("SolenoidDevRef"=w489:T13)  [unwired: 8 in, 1 out]
            n237 = Less Or Equal?(x=w498, y=1) -> (x <= y?=w497:bool)
          }
          n238 = call <vilib>:"WPI_SolenoidRefNum Registry Get.vi"("refnum name"="Piston 3") -> ("SolenoidDevRef"=w427:T13)  [unwired: 9 in, 1 out]
          n239 = while {
            tunnel: w427 -> [w462]
            tunnel: [w461] -> w426
            i -> [w463]
            stop <- w464 stop-if-true
            n240 = Increment(x=w463) -> (x+1=w465:i32)
            n241 = Wait (ms)(milliseconds to wait=u32 4500) -> ()  [unwired: 1 out]
            n242 = call-poly <vilib>:"WPI_SolenoidSet.vi"("Value"=WPI_SolenoidValue."Off", "SolenoidDevRef"=w462) -> ("SolenoidDevRef"=w461:T13)  [unwired: 8 in, 1 out]
            n243 = Less Or Equal?(x=w465, y=1) -> (x <= y?=w464:bool)
          }
          n244 = while {
            tunnel: w438 -> [w481]
            tunnel: w437 -> [w480]
            tunnel: [w479] -> w436
            tunnel: [w478] -> w435
            i -> [w485]
            stop <- w484 stop-if-true
            n245 = Increment(x=w485) -> (x+1=w486:i32)
            n246 = Wait (ms)(milliseconds to wait=u32 500) -> ()  [unwired: 1 out]
            n247 = call-poly <vilib>:"WPI_SolenoidSet.vi"("Value"=WPI_SolenoidValue."On", "SolenoidDevRef"=w481) -> ("SolenoidDevRef"=w478:T13)  [unwired: 8 in, 1 out]
            n248 = call-poly <vilib>:"WPI_SolenoidSet.vi"("Value"=WPI_SolenoidValue."On", "SolenoidDevRef"=w480) -> ("SolenoidDevRef"=w479:T13)  [unwired: 8 in, 1 out]
            n249 = Less Or Equal?(x=w486, y=1) -> (x <= y?=w484:bool)
          }
          n250 = while {
            tunnel: w426 -> [w454]
            i -> [w455]
            stop <- w456 stop-if-true
            n251 = Increment(x=w455) -> (x+1=w459:i32)
            n252 = Wait (ms)(milliseconds to wait=u32 500) -> ()  [unwired: 1 out]
            n253 = call-poly <vilib>:"WPI_SolenoidSet.vi"("Value"=WPI_SolenoidValue."On", "SolenoidDevRef"=w454) -> ()  [unwired: 8 in, 2 out]
            n254 = Less Or Equal?(x=w459, y=1) -> (x <= y?=w456:bool)
          }
          n255 = while {
            tunnel: w436 -> [w470]
            tunnel: w435 -> [w469]
            i -> [w474]
            stop <- w473 stop-if-true
            n256 = Increment(x=w474) -> (x+1=w475:i32)
            n257 = Wait (ms)(milliseconds to wait=u32 1000) -> ()  [unwired: 1 out]
            n258 = call-poly <vilib>:"WPI_SolenoidSet.vi"("Value"=WPI_SolenoidValue."Off", "SolenoidDevRef"=w469) -> ()  [unwired: 8 in, 2 out]
            n259 = call-poly <vilib>:"WPI_SolenoidSet.vi"("Value"=WPI_SolenoidValue."Off", "SolenoidDevRef"=w470) -> ()  [unwired: 8 in, 2 out]
            n260 = Less Or Equal?(x=w475, y=1) -> (x <= y?=w473:bool)
          }
          n261 = call <vilib>:"WPI_RobotDriveRefNum Registry Get.vi"("refnum name"="RobotDrive") -> ("RobotDriveDevRef"=w449:T7)  [unwired: 1 in, 9 out]
          n262 = call-poly <vilib>:"WPI_RobotDriveArcadeDrive.vi"("Y axis value"=-0.8 ("X axis value"), "X axis value"=0.0, "RobotDriveDevRef"=w449) -> ("Motor Values"=w453:dbl[], "RobotDriveDevRef"=w451:T7)  [unwired: 6 in, 1 out]
          n263 = call-poly <vilib>:"NT Write Value.vi"("Numeric Array"=w453, "Name"=w417) -> ()  [unwired: 9 in, 1 out]
          n264 = call <vilib>:"WPI_RobotDriveDelayAndUpdateSafety.vi"("Delay (s)"=T5 2.0, "RobotDriveDevRef"=w451) -> ("RobotDriveDevRef 2"=w430:T7)  [unwired: 8 in, 1 out]
          n265 = call-poly <vilib>:"WPI_RobotDriveArcadeDrive.vi"("Y axis value"=0.0 ("X axis value"), "X axis value"=-0.6, "RobotDriveDevRef"=w430) -> ("Motor Values"=w425:dbl[], "RobotDriveDevRef"=w431:T7)  [unwired: 6 in, 1 out]
          n266 = call-poly <vilib>:"NT Write Value.vi"("Numeric Array"=w425, "Name"=w417) -> ()  [unwired: 9 in, 1 out]
          n267 = call <vilib>:"WPI_RobotDriveDelayAndUpdateSafety.vi"("Delay (s)"=T5 0.55, "RobotDriveDevRef"=w431) -> ("RobotDriveDevRef 2"=w419:T7)  [unwired: 8 in, 1 out]
          n268 = call-poly <vilib>:"WPI_RobotDriveArcadeDrive.vi"("Y axis value"=-0.8 ("X axis value"), "X axis value"=0.0, "RobotDriveDevRef"=w419) -> ("Motor Values"=w424:dbl[], "RobotDriveDevRef"=w423:T7)  [unwired: 6 in, 1 out]
          n269 = call-poly <vilib>:"NT Write Value.vi"("Numeric Array"=w424, "Name"=w417) -> ()  [unwired: 9 in, 1 out]
          n270 = call <vilib>:"WPI_RobotDriveDelayAndUpdateSafety.vi"("Delay (s)"=T5 2.0, "RobotDriveDevRef"=w423) -> ("RobotDriveDevRef 2"=w418:T7)  [unwired: 8 in, 1 out]
          n271 = call-poly <vilib>:"WPI_RobotDriveArcadeDrive.vi"("Y axis value"=0.0 ("X axis value"), "X axis value"=0.0, "RobotDriveDevRef"=w418) -> ("Motor Values"=w452:dbl[], "RobotDriveDevRef"=w450:T7)  [unwired: 6 in, 1 out]
          n272 = call-poly <vilib>:"NT Write Value.vi"("Numeric Array"=w452, "Name"=w417) -> ()  [unwired: 9 in, 1 out]
          n273 = call <vilib>:"WPI_RobotDriveDelayAndUpdateSafety.vi"("Feed time (s)"=w429, "Delay (s)"=w429, "RobotDriveDevRef"=w450) -> ()  [unwired: 7 in, 2 out]
        }
        frame Default {
          w506 = "RobotDrive Motors" ("Name")
          # "CODE IS GOOD"
          # "stand still"
          # "Go Forwards"
          n274 = call <vilib>:"WPI_RobotDriveRefNum Registry Get.vi"("refnum name"="RobotDrive") -> ("RobotDriveDevRef"=w511:T7)  [unwired: 1 in, 9 out]
          n275 = call-poly <vilib>:"WPI_RobotDriveArcadeDrive.vi"("Y axis value"=-0.5 ("X axis value"), "X axis value"=0.0, "RobotDriveDevRef"=w511) -> ("Motor Values"=w516:dbl[], "RobotDriveDevRef"=w514:T7)  [unwired: 6 in, 1 out]
          n276 = call-poly <vilib>:"NT Write Value.vi"("Numeric Array"=w516, "Name"=w506) -> ()  [unwired: 9 in, 1 out]
          n277 = call <vilib>:"WPI_RobotDriveDelayAndUpdateSafety.vi"("Delay (s)"=T5 3.8, "RobotDriveDevRef"=w514) -> ("RobotDriveDevRef 2"=w513:T7)  [unwired: 8 in, 1 out]
          n278 = call <vilib>:"WPI_SolenoidRefNum Registry Get.vi"("refnum name"="Piston 3") -> ("SolenoidDevRef"=w501:T13)  [unwired: 9 in, 1 out]
          n279 = while {
            tunnel: w501 -> [w525]
            tunnel: [w524] -> w500
            i -> [w526]
            stop <- w527 stop-if-true
            n280 = Increment(x=w526) -> (x+1=w528:i32)
            n281 = Wait (ms)(milliseconds to wait=u32 4500) -> ()  [unwired: 1 out]
            n282 = call-poly <vilib>:"WPI_SolenoidSet.vi"("Value"=WPI_SolenoidValue."Off", "SolenoidDevRef"=w525) -> ("SolenoidDevRef"=w524:T13)  [unwired: 8 in, 1 out]
            n283 = Less Or Equal?(x=w528, y=1) -> (x <= y?=w527:bool)
          }
          n284 = call-poly <vilib>:"WPI_RobotDriveArcadeDrive.vi"("Y axis value"=0.0 ("X axis value"), "X axis value"=0.0, "RobotDriveDevRef"=w513) -> ("Motor Values"=w515:dbl[], "RobotDriveDevRef"=w512:T7)  [unwired: 6 in, 1 out]
          n285 = call-poly <vilib>:"NT Write Value.vi"("Numeric Array"=w515, "Name"=w506) -> ()  [unwired: 9 in, 1 out]
          n286 = call <vilib>:"WPI_RobotDriveDelayAndUpdateSafety.vi"("Delay (s)"=0.0, "RobotDriveDevRef"=w512) -> ()  [unwired: 8 in, 2 out]
          n287 = while {
            tunnel: w500 -> [w517]
            i -> [w518]
            stop <- w519 stop-if-true
            n288 = Increment(x=w518) -> (x+1=w522:i32)
            n289 = Wait (ms)(milliseconds to wait=u32 500) -> ()  [unwired: 1 out]
            n290 = call-poly <vilib>:"WPI_SolenoidSet.vi"("Value"=WPI_SolenoidValue."Off", "SolenoidDevRef"=w517) -> ()  [unwired: 8 in, 2 out]
            n291 = Less Or Equal?(x=w522, y=1) -> (x <= y?=w519:bool)
          }
        }
        frame "L" {
          w536 = "RobotDrive Motors" ("Name")
          # "CODE IS GOOD"
          # "stand still"
          # "Go Forwards"
          n292 = call <vilib>:"WPI_RobotDriveRefNum Registry Get.vi"("refnum name"="RobotDrive") -> ("RobotDriveDevRef"=w543:T7)  [unwired: 1 in, 9 out]
          n293 = call <vilib>:"WPI_SolenoidRefNum Registry Get.vi"("refnum name"="Piston 3") -> ("SolenoidDevRef"=w533:T13)  [unwired: 9 in, 1 out]
          n294 = call-poly <vilib>:"WPI_RobotDriveArcadeDrive.vi"("Y axis value"=-0.8 ("X axis value"), "X axis value"=0.0, "RobotDriveDevRef"=w543) -> ("Motor Values"=w548:dbl[], "RobotDriveDevRef"=w546:T7)  [unwired: 6 in, 1 out]
          n295 = while {
            tunnel: w533 -> [w557]
            tunnel: [w556] -> w532
            i -> [w558]
            stop <- w559 stop-if-true
            n296 = Increment(x=w558) -> (x+1=w560:i32)
            n297 = Wait (ms)(milliseconds to wait=u32 4000) -> ()  [unwired: 1 out]
            n298 = call-poly <vilib>:"WPI_SolenoidSet.vi"("Value"=WPI_SolenoidValue."Off", "SolenoidDevRef"=w557) -> ("SolenoidDevRef"=w556:T13)  [unwired: 8 in, 1 out]
            n299 = Less Or Equal?(x=w560, y=1) -> (x <= y?=w559:bool)
          }
          n300 = call-poly <vilib>:"NT Write Value.vi"("Numeric Array"=w548, "Name"=w536) -> ()  [unwired: 9 in, 1 out]
          n301 = call <vilib>:"WPI_RobotDriveDelayAndUpdateSafety.vi"("Delay (s)"=T5 2.0, "RobotDriveDevRef"=w546) -> ("RobotDriveDevRef 2"=w545:T7)  [unwired: 8 in, 1 out]
          n302 = call-poly <vilib>:"WPI_RobotDriveArcadeDrive.vi"("Y axis value"=0.0 ("X axis value"), "X axis value"=0.0, "RobotDriveDevRef"=w545) -> ("Motor Values"=w547:dbl[], "RobotDriveDevRef"=w544:T7)  [unwired: 6 in, 1 out]
          n303 = while {
            tunnel: w532 -> [w549]
            i -> [w550]
            stop <- w551 stop-if-true
            n304 = Increment(x=w550) -> (x+1=w554:i32)
            n305 = Wait (ms)(milliseconds to wait=u32 500) -> ()  [unwired: 1 out]
            n306 = call-poly <vilib>:"WPI_SolenoidSet.vi"("Value"=WPI_SolenoidValue."Off", "SolenoidDevRef"=w549) -> ()  [unwired: 8 in, 2 out]
            n307 = Less Or Equal?(x=w554, y=1) -> (x <= y?=w551:bool)
          }
          n308 = call-poly <vilib>:"NT Write Value.vi"("Numeric Array"=w547, "Name"=w536) -> ()  [unwired: 9 in, 1 out]
          n309 = call <vilib>:"WPI_RobotDriveDelayAndUpdateSafety.vi"("Delay (s)"=0.0, "RobotDriveDevRef"=w544) -> ()  [unwired: 8 in, 2 out]
        }
      }
    }
  }
